vi "Climb_Off_Platform.vi"(1 "Startup":bool) -> (2 "Elevator_Break_State":T1=enum."On", 3 "Back_Lift_State":T1=enum."On", 4 "Swerve_X":dbl format="%#_13g", 6 "Back_Lift_Velocity":dbl format="%#_13g", 8 "Front_Lift_Velocity":dbl format="%#_13g", 10 "Back_Elevator_Wheels":dbl format="%#_13g", 12 "Completed":bool, 14 "Reint":bool)   [LabVIEW 2018]
uses:
  <vilib>/Rock Robotics/WPI/Solenoid/WPI_SolenoidValue.ctl
  Autonomous Utilities/Command_Execution_State.ctl
  Auto_Climb_Off_Platform_States.ctl
  Global_Variables/Sensor_Values.vi
  Global_Variables/Climb_Globals.vi
  Global_Variables/Elevator_Globals.vi
panel:
  in  "Elevator_Gain":dbl=0.00012
  in  "Front_Lift_Down_Dist":dbl
  in  "Back_Lift_Time_Off_Platform":dbl
  in  "Swerve_Distance_Off_Platform":dbl
  in  "Between_Lift_Acceptable_Error":dbl
  in  "Elevator_Gain":dbl=0.00012
  in  "Elevator_Between_Gain":dbl=0.00013
  in  "Back_Lift_Distance":dbl
  in  "Back_Lift_Gain":dbl=0.00012
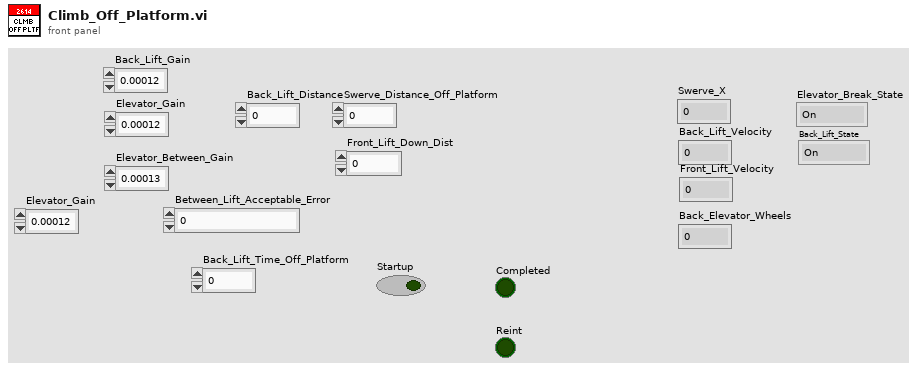
[diagram p1: front panel]
types:
  T1 = typedef "WPI_SolenoidValue.ctl" = enum16{"Off", "On", "Forward", "Reverse"}
  T2 = typedef "Command_Execution_State.ctl" = enum16{"Initialize", "Execute", "Finish"}
  T3 = typedef "Auto_Climb_Off_Platform_States.ctl" = enum16{"Back_Lift_Extend", "Swerve_and_Back_Reverse", "Front_Lift_Extend", "Back_Lift_Wheels_Reverse", "Lifts_Retract"}
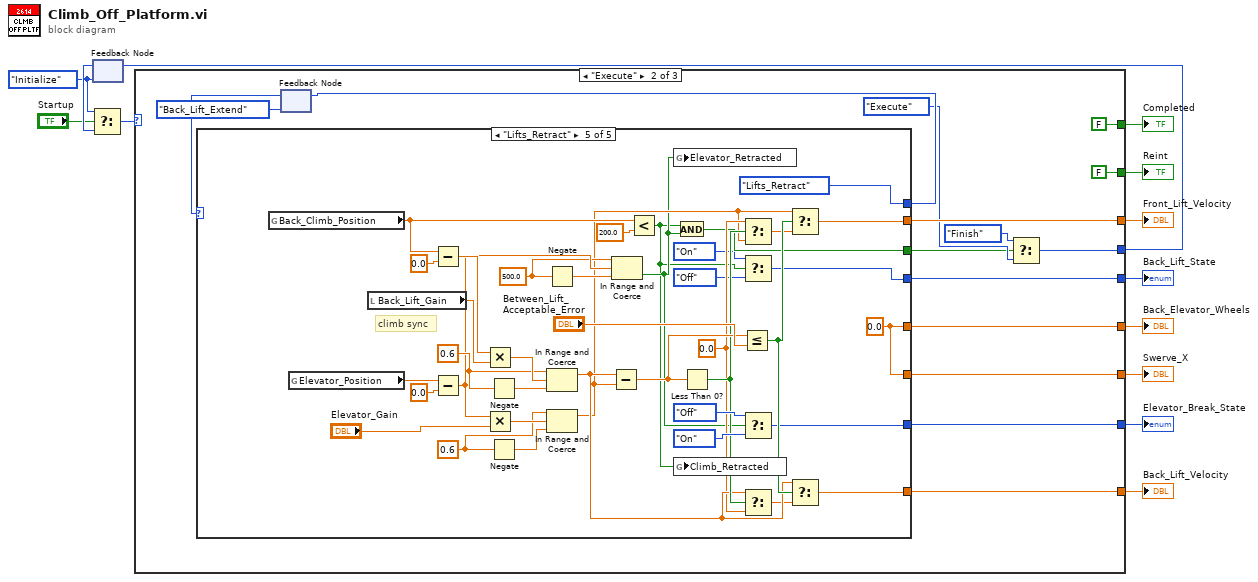
[diagram p0: block diagram]
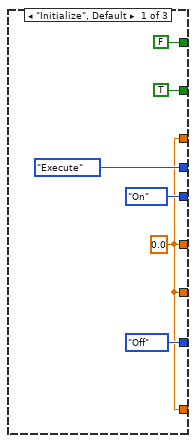
[diagram p2: hidden frame]
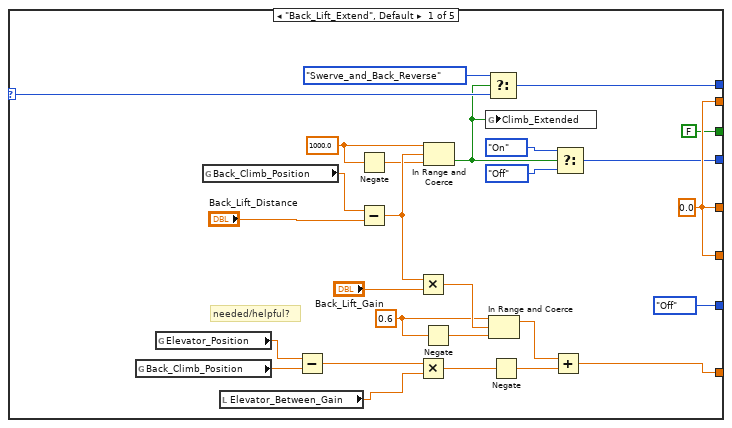
[diagram p3: hidden frame]
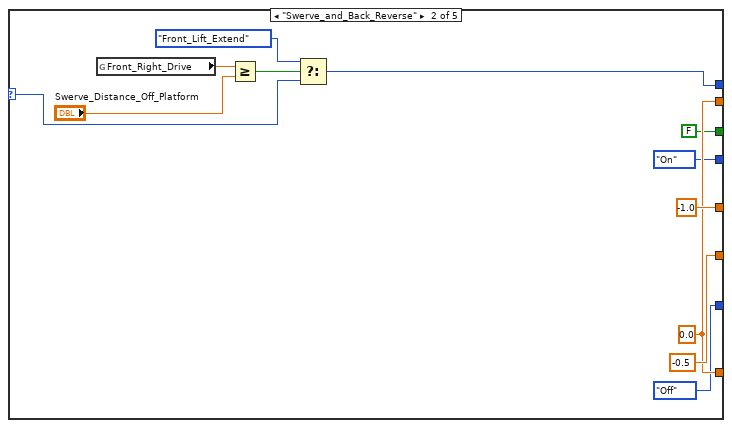
[diagram p4: hidden frame]
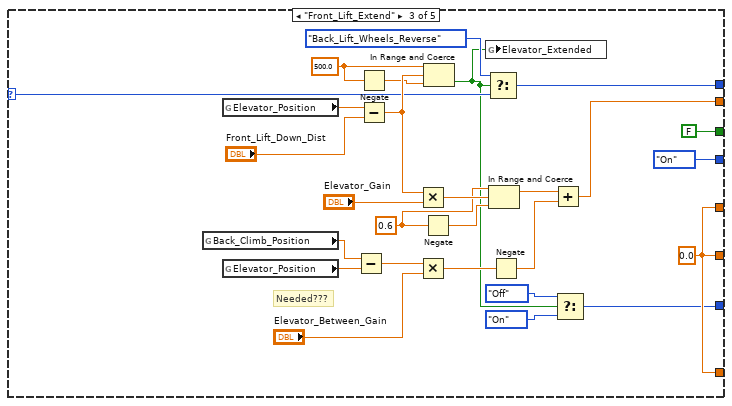
[diagram p5: hidden frame]
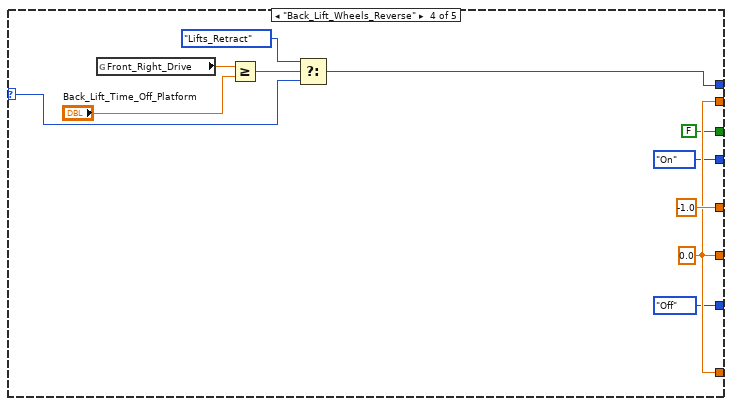
[diagram p6: hidden frame]
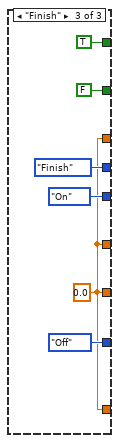
[diagram p7: hidden frame]
diagram:
  w7 = Command_Execution_State."Initialize" ("Play State")
  n1 = feedback #1(w7) -> (w11:T2)
  n2 = Select(t=w7, s="Startup", f=w11) -> (s? t:f=w13:T2)
  n3 = case shown="\"Execute\"" w13 {
    tunnel: [Command_Execution_State."Execute" ("Play State") w23 Command_Execution_State."Finish" ("Play State")] -> w12
    tunnel: [FALSE FALSE TRUE] -> w10
    tunnel: [TRUE FALSE FALSE] -> w8
    tunnel: [w14 w31 w151] -> w6
    tunnel: [w14 w32 w151] -> w5
    tunnel: [w14 w30 w151] -> w4
    tunnel: [w14 w29 w151] -> w3
    tunnel: [WPI_SolenoidValue."On" ("Value") w21 WPI_SolenoidValue."On" ("Value")] -> w1
    tunnel: [WPI_SolenoidValue."Off" ("Value") w20 WPI_SolenoidValue."Off" ("Value")] -> w2
    frame "Initialize", Default {
      w14 = 0.0
    }
    frame "Execute" {
      n4 = feedback #2(Auto_Climb_Off_Platform_States."Back_Lift_Extend" ("Climb_Control_Type")) -> (w27:T3)
      n5 = case shown="\"Lifts_Retract\"" w27 {
        selector: w27 -> [w44 w68 w79 w104 _]
        tunnel: [w46 w71 w100 w110 w132] -> w32
        tunnel: [w45 -0.5 w100 w110 w128] -> w31
        tunnel: [w45 -1.0 w100 -1.0 w128] -> w30
        tunnel: [w45 w71 w82 w110 w129] -> w29
        tunnel: [w42 w69 w80 w105 Auto_Climb_Off_Platform_States."Lifts_Retract" ("Climb_Control_Type")] -> w26
        tunnel: [FALSE FALSE FALSE FALSE w119] -> w22
        tunnel: [w37 WPI_SolenoidValue."On" ("Value") WPI_SolenoidValue."On" ("Value") WPI_SolenoidValue."On" ("Value") w114] -> w21
        tunnel: [WPI_SolenoidValue."Off" ("Value") WPI_SolenoidValue."Off" ("Value") w76 WPI_SolenoidValue."Off" ("Value") w118] -> w20
        frame "Back_Lift_Extend", Default {
          w45 = 0.0
          w49 = 1000.0 ("upper limit")
          w48 = 0.6 ("upper limit")
          # "needed/helpful?"
          n6 = global read "Sensor_Values.vi" "Back_Climb_Position"() -> (w53:dbl)
          n7 = global read "Sensor_Values.vi" "Elevator_Position"() -> (w52:dbl)
          n8 = global read "Sensor_Values.vi" "Back_Climb_Position"() -> (w59:dbl)
          n9 = local read "Elevator_Between_Gain"() -> (w35:dbl)
          n10 = Subtract(x=w52, y=w53) -> (x-y=w51:dbl)
          n11 = Negate(x=w49) -> (-x=w60:dbl)
          n12 = Subtract(x=w59, y="Back_Lift_Distance") -> (x-y=w61:dbl)
          n13 = Multiply(x=w61, y="Back_Lift_Gain") -> (x*y=w56:dbl)
          n14 = Multiply(x=w51, y=w35) -> (x*y=w50:dbl)
          n15 = Negate(x=w48) -> (-x=w55:dbl)
          n16 = In Range and Coerce(upper limit=w49, x=w61, lower limit=w60) -> (In Range?=w40:bool)  [unwired: 1 out]
          n17 = global write "Climb_Globals.vi" "Climb_Extended"(w40) -> ()
          n18 = Select(t=Auto_Climb_Off_Platform_States."Swerve_and_Back_Reverse" ("Climb_Control_Type"), s=w40, f=w44) -> (s? t:f=w42:T3)
          n19 = In Range and Coerce(upper limit=w48, x=w56, lower limit=w55) -> (coerced(x)=w58:dbl)  [unwired: 1 out]
          n20 = Negate(x=w50) -> (-x=w54:dbl)
          n21 = Add(x=w58, y=w54) -> (x+y=w46:dbl)
          n22 = Select(t=WPI_SolenoidValue."On" ("Back_Lift_State"), s=w40, f=WPI_SolenoidValue."Off" ("Back_Lift_State")) -> (s? t:f=w37:T1)
        }
        frame "Swerve_and_Back_Reverse" {
          w71 = 0.0
          n23 = global read "Sensor_Values.vi" "Front_Right_Drive"() -> (w67:dbl)
          n24 = Greater Or Equal?(x=w67, y="Swerve_Distance_Off_Platform") -> (x >= y?=w65:bool)
          n25 = Select(t=Auto_Climb_Off_Platform_States."Front_Lift_Extend" ("Climb_Control_Type"), s=w65, f=w68) -> (s? t:f=w69:T3)
        }
        frame "Front_Lift_Extend" {
          w84 = 500.0 ("upper limit")
          w87 = 0.6 ("upper limit")
          w100 = 0.0
          # "Needed???"
          n26 = global read "Sensor_Values.vi" "Back_Climb_Position"() -> (w88:dbl)
          n27 = global read "Sensor_Values.vi" "Elevator_Position"() -> (w95:dbl)
          n28 = global read "Sensor_Values.vi" "Elevator_Position"() -> (w89:dbl)
          n29 = Subtract(x=w88, y=w89) -> (x-y=w90:dbl)
          n30 = Negate(x=w84) -> (-x=w85:dbl)
          n31 = Subtract(x=w95, y="Front_Lift_Down_Dist") -> (x-y=w99:dbl)
          n32 = Multiply(x=w99, y="Elevator_Gain") -> (x*y=w96:dbl)
          n33 = Multiply(x=w90, y="Elevator_Between_Gain") -> (x*y=w92:dbl)
          n34 = Negate(x=w87) -> (-x=w94:dbl)
          n35 = In Range and Coerce(upper limit=w84, x=w99, lower limit=w85) -> (In Range?=w78:bool)  [unwired: 1 out]
          n36 = global write "Elevator_Globals.vi" "Elevator_Extended"(w78) -> ()
          n37 = Select(t=Auto_Climb_Off_Platform_States."Back_Lift_Wheels_Reverse" ("Climb_Control_Type"), s=w78, f=w79) -> (s? t:f=w80:T3)
          n38 = In Range and Coerce(upper limit=w87, x=w96, lower limit=w94) -> (coerced(x)=w93:dbl)  [unwired: 1 out]
          n39 = Negate(x=w92) -> (-x=w98:dbl)
          n40 = Add(x=w93, y=w98) -> (x+y=w82:dbl)
          n41 = Select(t=WPI_SolenoidValue."Off" ("Value"), s=w78, f=WPI_SolenoidValue."On" ("Value")) -> (s? t:f=w76:T1)
        }
        frame "Back_Lift_Wheels_Reverse" {
          w110 = 0.0
          n42 = global read "Sensor_Values.vi" "Front_Right_Drive"() -> (w108:dbl)
          n43 = Greater Or Equal?(x=w108, y="Back_Lift_Time_Off_Platform") -> (x >= y?=w106:bool)
          n44 = Select(t=Auto_Climb_Off_Platform_States."Lifts_Retract" ("Climb_Control_Type"), s=w106, f=w104) -> (s? t:f=w105:T3)
        }
        frame "Lifts_Retract" {
          w124 = 0.0
          w128 = 0.0
          w134 = 500.0 ("upper limit")
          w139 = 0.6 ("upper limit")
          w145 = 0.6 ("upper limit")
          # "climb sync"
          n45 = global read "Sensor_Values.vi" "Back_Climb_Position"() -> (w143:dbl)
          n46 = global read "Sensor_Values.vi" "Elevator_Position"() -> (w140:dbl)
          n47 = local read "Back_Lift_Gain"() -> (w149:dbl)
          n48 = Subtract(x=w143, y=0.0) -> (x-y=w150:dbl)
          n49 = Subtract(x=w140, y=0.0) -> (x-y=w135:dbl)
          n50 = Multiply(x=w150, y=w149) -> (x*y=w148:dbl)
          n51 = Multiply(x=w135, y="Elevator_Gain") -> (x*y=w141:dbl)
          n52 = Negate(x=w145) -> (-x=w147:dbl)
          n53 = Negate(x=w139) -> (-x=w142:dbl)
          n54 = Negate(x=w134) -> (-x=w133:dbl)
          n55 = In Range and Coerce(upper limit=w145, x=w148, lower limit=w147) -> (coerced(x)=w125:dbl)  [unwired: 1 out]
          n56 = In Range and Coerce(upper limit=w139, x=w141, lower limit=w142) -> (coerced(x)=w123:dbl)  [unwired: 1 out]
          n57 = Subtract(x=w125, y=w123) -> (x-y=w127:dbl)
          n58 = In Range and Coerce(upper limit=w134, x=w135, lower limit=w133) -> (In Range?=w120:bool)  [unwired: 1 out]
          n59 = Less?(x=w143, y=200.0) -> (x < y?=w115:bool)
          n60 = global write "Elevator_Globals.vi" "Elevator_Retracted"(w120) -> ()
          n61 = global write "Climb_Globals.vi" "Climb_Retracted"(w115) -> ()
          n62 = And(x=w115, y=w120) -> (x .and. y?=w119:bool)
          n63 = Less Than 0?(x=w127) -> (x < 0?=w126:bool)
          n64 = Less Or Equal?(x=w127, y="Between_Lift_Acceptable_Error") -> (x <= y?=w131:bool)
          n65 = Select(t=w124, s=w126, f=w123) -> (s? t:f=w122:dbl)
          n66 = Select(t=WPI_SolenoidValue."On" ("Back_Lift_State"), s=w115, f=WPI_SolenoidValue."Off" ("Back_Lift_State")) -> (s? t:f=w114:T1)
          n67 = Select(t=WPI_SolenoidValue."Off" ("Value"), s=w120, f=WPI_SolenoidValue."On" ("Value")) -> (s? t:f=w118:T1)
          n68 = Select(t=w125, s=w126, f=w124) -> (s? t:f=w121:dbl)
          n69 = Select(t=w123, s=w131, f=w122) -> (s? t:f=w129:dbl)
          n70 = Select(t=w125, s=w131, f=w121) -> (s? t:f=w132:dbl)
        }
      }
      n71 = feedback-in #2(w26) -> ()
      n72 = Select(t=Command_Execution_State."Finish" ("Play State"), s=w22, f=Command_Execution_State."Execute" ("Play State")) -> (s? t:f=w23:T2)
    }
    frame "Finish" {
      w151 = 0.0
    }
  }
  "Completed" <- w10
  "Reint" <- w8
  "Back_Elevator_Wheels" <- w4
  "Back_Lift_Velocity" <- w5
  "Swerve_X" <- w6
  "Front_Lift_Velocity" <- w3
  "Elevator_Break_State" <- w2
  "Back_Lift_State" <- w1
  n73 = feedback-in #1(w12) -> ()
